vi "CRYSet Control Caption and Text.vi"(8 "Tooltip":string, 9 "Control Type":string, 10 "Caption":string, 11 "Control reference In":refnum<vi>) -> (3 "Control reference out":refnum<vi>)   [LabVIEW 2013]
uses:
  CRYMainGlobal.vi
panel:
  out "error out":errorcluster
  in  "Interpret as Unicode (T)":bool
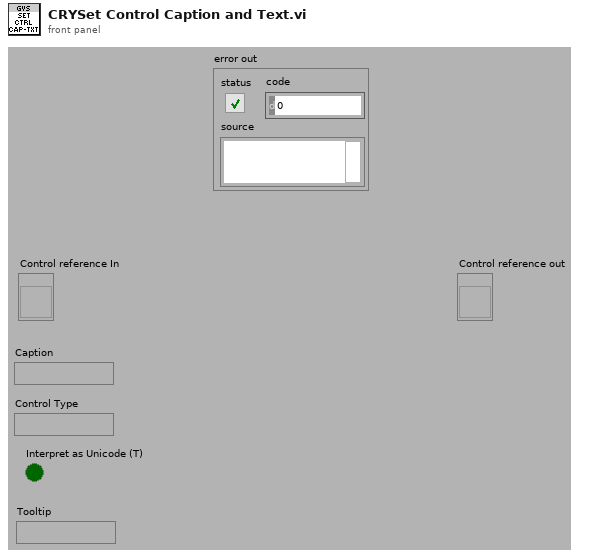
[diagram p1: front panel]
types:
  T1 = enum32{"English", "Chinese", "Korean", "Japanese", "Russian", "Chinese traditional"}
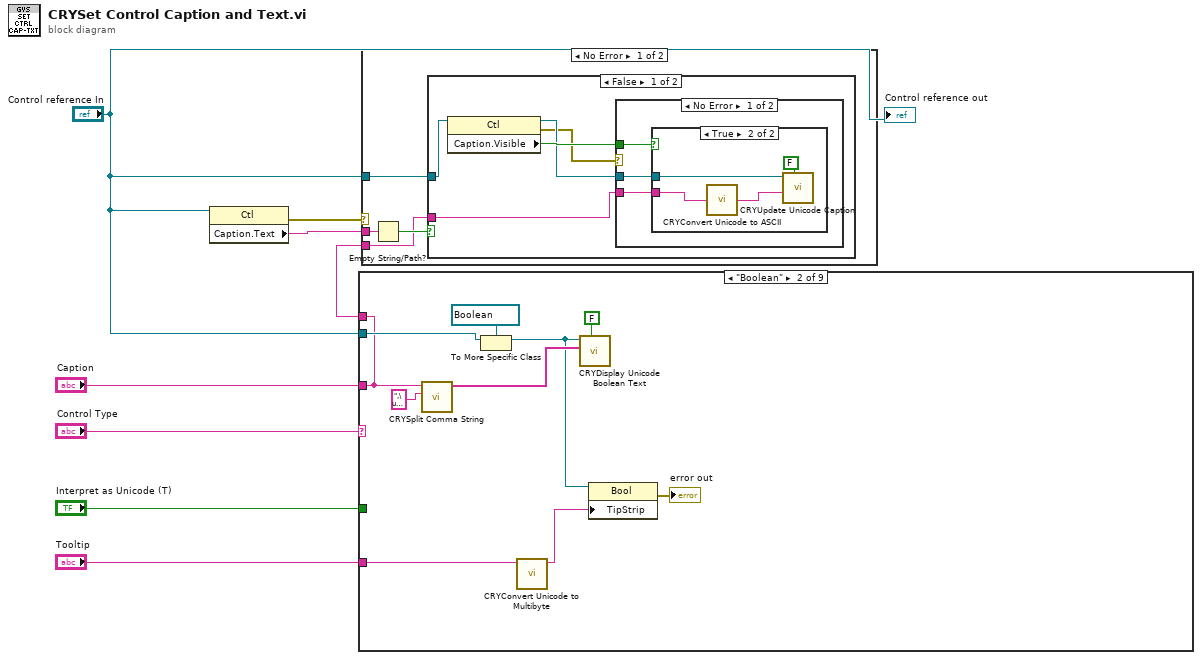
[diagram p0: block diagram]
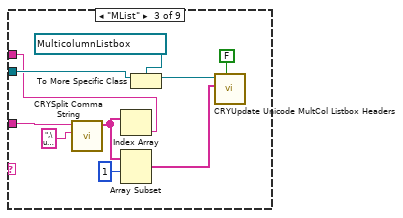
[diagram p7: hidden frame]
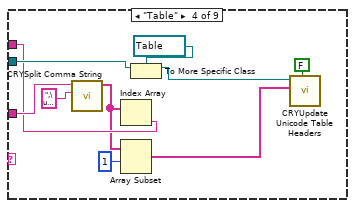
[diagram p8: hidden frame]
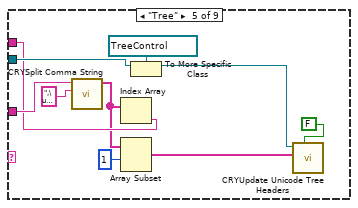
[diagram p9: hidden frame]
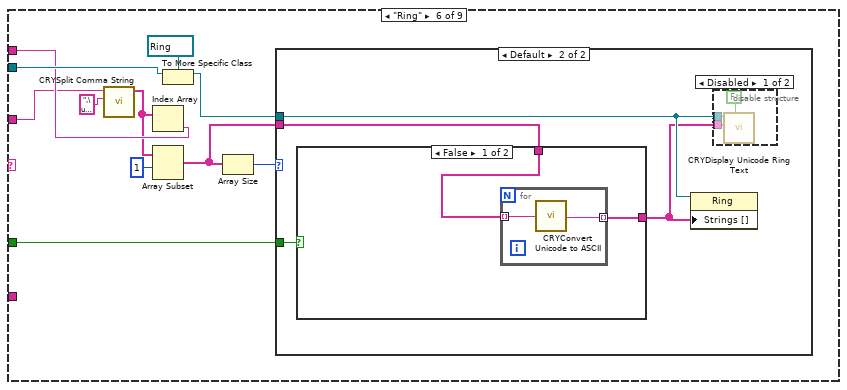
[diagram p10: hidden frame]
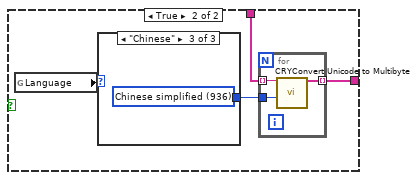
[diagram p12: hidden frame]
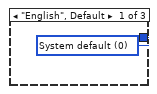
[diagram p13: hidden frame]
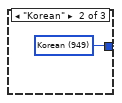
[diagram p14: hidden frame]
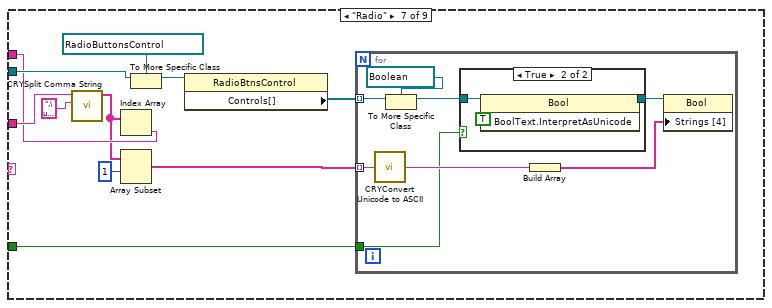
[diagram p16: hidden frame]
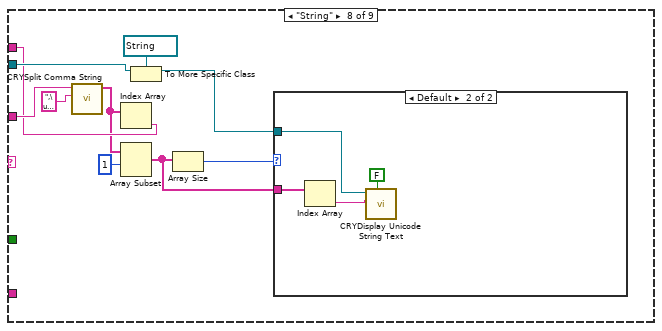
[diagram p18: hidden frame]
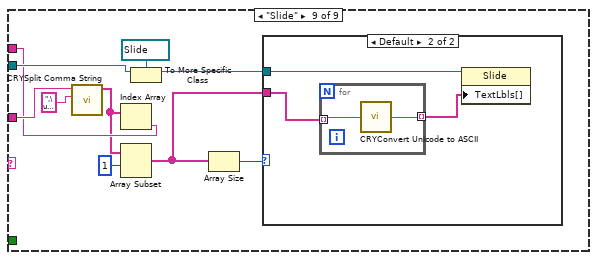
[diagram p20: hidden frame]
diagram:
  n1 = property class="Ctl"(reference="Control reference In") -> (error out=w3:errorcluster, "Caption.Text"=w8:string)  [unwired: 1 in, 1 out]
  n2 = case shown="\"Boolean\"" "Control Type" {
    tunnel: "Control reference In" -> [_ w18 w29 w39 w49 w60 w92 w114 w128]
    tunnel: "Caption" -> [w9 w14 w27 w38 w48 w51 w91 w113 w127]
    tunnel: [w9 w14 w23 w36 w46 w59 w90 w112 w125] -> w4
    tunnel: "Interpret as Unicode (T)" -> [_ _ _ _ _ w50 w82 _ _]
    tunnel: "Tooltip" -> [_ w11 _ _ _ _ _ _ _]
    frame Default {
    }
    frame "Boolean" {
      n3 = call "CRYSplit Comma String.vi"("sSplit Letter"=",\u0000" ("Label.Text"), "sData Out"=w14) -> ("Array"=w16:string[])  [unwired: 9 in]
      n4 = To More Specific Class(target class=refnum<vi> refnum ("Tab Control"), reference=w18) -> (specific class reference=w13:refnum<vi>)  [unwired: 1 in, 1 out]
      n5 = call "CRYConvert Unicode to Multibyte.vi"("Unicode String"=w11) -> ("Multibyte string"=w10:string)  [unwired: 9 in, 1 out]
      n6 = call "CRYDisplay Unicode Boolean Text.vi"("Interpret as Unicode (T)"=FALSE, "Boolean Texts [4]"=w16, "Boolean Reference"=w13) -> ()  [unwired: 5 in, 2 out]
      n7 = property class="Bool"(reference=w13, "TipStrip"=w10) -> (error out=→"error out":errorcluster)  [unwired: 1 in, 1 out]
    }
    frame "MList" {
      n8 = call "CRYSplit Comma String.vi"("sSplit Letter"=",\u0000" ("Label.Text"), "sData Out"=w27) -> ("Array"=w22:string[])  [unwired: 9 in]
      n9 = Index Array(array=w22) -> (element=w23:string)  [unwired: 1 in]
      n10 = Array Subset(array=w22, index=1) -> (w20:string[])  [unwired: 1 in]
      n11 = To More Specific Class(target class=refnum<vi> refnum ("Multicolumn Listbox Ref"), reference=w29) -> (specific class reference=w24:refnum<vi>)  [unwired: 1 in, 1 out]
      n12 = call "CRYUpdate Unicode MultCol Listbox Headers.vi"("Interpret as Unicode (T)"=FALSE, "Column Headers[]"=w20, "Multicolumn Listbox Ref"=w24) -> ()  [unwired: 7 in, 2 out]
    }
    frame "Table" {
      n13 = call "CRYSplit Comma String.vi"("sSplit Letter"=",\u0000" ("Label.Text"), "sData Out"=w38) -> ("Array"=w35:string[])  [unwired: 9 in]
      n14 = Index Array(array=w35) -> (element=w36:string)  [unwired: 1 in]
      n15 = Array Subset(array=w35, index=1) -> (w32:string[])  [unwired: 1 in]
      n16 = To More Specific Class(target class=refnum<vi> refnum ("Table Ref"), reference=w39) -> (specific class reference=w31:refnum<vi>)  [unwired: 1 in, 1 out]
      n17 = call "CRYUpdate Unicode Table Headers.vi"("Interpret as Unicode (T)"=FALSE, "Column Headers[]"=w32, "Table Ref"=w31) -> ()  [unwired: 7 in, 2 out]
    }
    frame "Tree" {
      n18 = call "CRYSplit Comma String.vi"("sSplit Letter"=",\u0000" ("Label.Text"), "sData Out"=w48) -> ("Array"=w45:string[])  [unwired: 9 in]
      n19 = Index Array(array=w45) -> (element=w46:string)  [unwired: 1 in]
      n20 = Array Subset(array=w45, index=1) -> (w43:string[])  [unwired: 1 in]
      n21 = To More Specific Class(target class=refnum<vi> refnum ("Table Ref"), reference=w49) -> (specific class reference=w40:refnum<vi>)  [unwired: 1 in, 1 out]
      n22 = call "CRYUpdate Unicode Tree Headers.vi"("Interpret as Unicode (T)"=FALSE, "Column Headers[]"=w43, "Tree Ref"=w40) -> ()  [unwired: 7 in, 2 out]
    }
    frame "Ring" {
      n23 = call "CRYSplit Comma String.vi"("sSplit Letter"=",\u0000" ("Label.Text"), "sData Out"=w51) -> ("Array"=w57:string[])  [unwired: 9 in]
      n24 = Index Array(array=w57) -> (element=w59:string)  [unwired: 1 in]
      n25 = Array Subset(array=w57, index=1) -> (w53:string[])  [unwired: 1 in]
      n26 = To More Specific Class(target class=refnum<vi> refnum ("Ring Control Ref"), reference=w60) -> (specific class reference=w54:refnum<vi>)  [unwired: 1 in, 1 out]
      n27 = Array Size(array=w53) -> (size(s)=w52:i32)
      n28 = case shown="Default" w52 {
        tunnel: w54 -> [_ w63]
        tunnel: w53 -> [_ w64]
        tunnel: w50 -> [_ w61]
        frame 0 {
        }
        frame Default {
          n29 = case shown="False" w61 {
            tunnel: w64 -> [w66 w70]
            tunnel: [w65 w69] -> w62
            frame False {
              n30 = for {
                tunnel: w66 -> [w68] mode=indexing
                tunnel: [w67] -> w65 mode=indexing
                n31 = call "CRYConvert Unicode to ASCII.vi"("Unicode"=w68) -> ("ASCII"=w67:string)  [unwired: 4 in]
              }
            }
            frame True {
              n32 = global read "CRYMainGlobal.vi" "Language"() -> (w72:T1)
              n33 = case shown="\"Chinese\"" w72 {
                tunnel: [w76 w77 w78] -> w71
                frame "English", Default {
                  w76 = u32 0 items=["System default"=0, "Latin-1"=1252, "Japanese"=932, "Korean"=949, "Chinese simplified"=936, "Chinese traditional"=950, "Central Europe"=1250, "Cyrillic"=1251, "Greek"=1253, "Turkish"=1254, "Hebrew"=1255, "Arabic"=1256, "Baltic"=1257, "Thai"=874, "Vietnamese"=783, "UTF8"=65001, "UTF-7"=65000] ("Code Page")
                }
                frame "Korean" {
                  w77 = u32 949 items=["System default"=0, "Latin-1"=1252, "Japanese"=932, "Korean"=949, "Chinese simplified"=936, "Chinese traditional"=950, "Central Europe"=1250, "Cyrillic"=1251, "Greek"=1253, "Turkish"=1254, "Hebrew"=1255, "Arabic"=1256, "Baltic"=1257, "Thai"=874, "Vietnamese"=783, "UTF8"=65001, "UTF-7"=65000] ("Code Page")
                }
                frame "Chinese" {
                  w78 = u32 936 items=["System default"=0, "Latin-1"=1252, "Japanese"=932, "Korean"=949, "Chinese simplified"=936, "Chinese traditional"=950, "Central Europe"=1250, "Cyrillic"=1251, "Greek"=1253, "Turkish"=1254, "Hebrew"=1255, "Arabic"=1256, "Baltic"=1257, "Thai"=874, "Vietnamese"=783, "UTF8"=65001, "UTF-7"=65000] ("Code Page")
                }
              }
              n34 = for {
                tunnel: w70 -> [w75] mode=indexing
                tunnel: [w74] -> w69 mode=indexing
                tunnel: w71 -> [w73]
                n35 = call "CRYConvert Unicode to Multibyte.vi"("Code Page"=w73, "Unicode String"=w75) -> ("Multibyte string"=w74:string)  [unwired: 8 in, 1 out]
              }
            }
          }
          n36 = property class="Ring"(reference=w63, "Strings []"=w62) -> ()  [unwired: 1 in, 2 out]
          n37 = disable-structure shown="Disabled" {
            disable-tunnel: w63 -> [w80 _]
            disable-tunnel: w62 -> [w79 _]
            frame Disabled {
              n38 = call "CRYDisplay Unicode Ring Text.vi"("Interpret as Unicode (T)"=FALSE, "Ring Texts"=w79, "Ring Control Ref"=w80) -> ()  [unwired: 5 in, 2 out]
            }
            frame Enabled {
            }
          }
        }
      }
    }
    frame "Radio" {
      n39 = call "CRYSplit Comma String.vi"("sSplit Letter"=",\u0000" ("Label.Text"), "sData Out"=w91) -> ("Array"=w88:string[])  [unwired: 9 in]
      n40 = Index Array(array=w88) -> (element=w90:string)  [unwired: 1 in]
      n41 = Array Subset(array=w88, index=1) -> (w83:string[])  [unwired: 1 in]
      n42 = To More Specific Class(target class=refnum<vi> refnum ("Radio Buttons"), reference=w92) -> (specific class reference=w85:refnum<vi>)  [unwired: 1 in, 1 out]
      n43 = property class="RadioBtnsControl"(reference=w85) -> ("Controls[]"=w84:refnum<vi>[])  [unwired: 1 in, 2 out]
      n44 = for {
        tunnel: w84 -> [w99] mode=indexing
        tunnel: w83 -> [w95] mode=indexing
        tunnel: w82 -> [w93]
        n45 = call "CRYConvert Unicode to ASCII.vi"("Unicode"=w95) -> ("ASCII"=w94:string)  [unwired: 4 in]
        n46 = To More Specific Class(target class=refnum<vi> refnum ("Radio Selection 2"), reference=w99) -> (specific class reference=w97:refnum<vi>)  [unwired: 1 in, 1 out]
        n47 = case shown="True" w93 {
          tunnel: w97 -> [w101 w104]
          tunnel: [w101 w102] -> w96
          frame False {
          }
          frame True {
            n48 = property class="Bool"(reference=w104, "BoolText.InterpretAsUnicode"=TRUE ("Boolean Text.Interpret As Unicode")) -> (reference out=w102:refnum<vi>)  [unwired: 1 in, 1 out]
          }
        }
        n49 = Build Array(w94) -> (w98:string[])
        n50 = property class="Bool"(reference=w96, "Strings [4]"=w98) -> ()  [unwired: 1 in, 2 out]
      }
    }
    frame "String" {
      n51 = call "CRYSplit Comma String.vi"("sSplit Letter"=",\u0000" ("Label.Text"), "sData Out"=w113) -> ("Array"=w110:string[])  [unwired: 9 in]
      n52 = Index Array(array=w110) -> (element=w112:string)  [unwired: 1 in]
      n53 = Array Subset(array=w110, index=1) -> (w105:string[])  [unwired: 1 in]
      n54 = To More Specific Class(target class=refnum<vi> refnum ("Radio Buttons"), reference=w114) -> (specific class reference=w106:refnum<vi>)  [unwired: 1 in, 1 out]
      n55 = Array Size(array=w105) -> (size(s)=w107:i32)
      n56 = case shown="Default" w107 {
        tunnel: w106 -> [_ w117]
        tunnel: w105 -> [_ w118]
        frame 0 {
        }
        frame Default {
          n57 = Index Array(array=w118) -> (element=w116:string)  [unwired: 1 in]
          n58 = call "CRYDisplay Unicode String Text.vi"("Interpret as Unicode (T)"=FALSE, "String Value"=w116, "String Control Reference"=w117) -> ()  [unwired: 5 in, 2 out]
        }
      }
    }
    frame "Slide" {
      n59 = call "CRYSplit Comma String.vi"("sSplit Letter"=",\u0000" ("Label.Text"), "sData Out"=w127) -> ("Array"=w124:string[])  [unwired: 9 in]
      n60 = Index Array(array=w124) -> (element=w125:string)  [unwired: 1 in]
      n61 = Array Subset(array=w124, index=1) -> (w120:string[])  [unwired: 1 in]
      n62 = To More Specific Class(target class=refnum<vi> refnum ("Scale 2"), reference=w128) -> (specific class reference=w121:refnum<vi>)  [unwired: 1 in, 1 out]
      n63 = Array Size(array=w120) -> (size(s)=w119:i32)
      n64 = case shown="Default" w119 {
        tunnel: w121 -> [_ w131]
        tunnel: w120 -> [_ w130]
        frame 0 {
        }
        frame Default {
          n65 = for {
            tunnel: w130 -> [w133] mode=indexing
            tunnel: [w132] -> w129 mode=indexing
            n66 = call "CRYConvert Unicode to ASCII.vi"("Unicode"=w133) -> ("ASCII"=w132:string)  [unwired: 4 in]
          }
          n67 = property class="Slide"(reference=w131, "TextLbls[]"=w129) -> ()  [unwired: 1 in, 2 out]
        }
      }
    }
  }
  n68 = case shown="No Error" w3 {
    tunnel: w8 -> [w136 _]
    tunnel: "Control reference In" -> [w135 _]
    tunnel: w4 -> [w134 _]
    frame No Error {
      n69 = Empty String/Path?(string/path=w136) -> (empty?=w137:bool)
      n70 = case shown="False" w137 {
        tunnel: w135 -> [w140 _]
        tunnel: w134 -> [w139 _]
        frame False {
          n71 = property class="Ctl"(reference=w140) -> (error out=w138:errorcluster, "Caption.Visible"=w141:bool)  [unwired: 1 in, 1 out]
          n72 = case shown="No Error" w138 {
            tunnel: w141 -> [w144 _]
            tunnel: w140 -> [w143 _]
            tunnel: w139 -> [w142 _]
            frame No Error {
              n73 = case shown="True" w144 {
                tunnel: w143 -> [_ w148]
                tunnel: w142 -> [_ w146]
                frame False {
                }
                frame True {
                  n74 = call "CRYConvert Unicode to ASCII.vi"("Unicode"=w146) -> ("ASCII"=w145:string)  [unwired: 4 in]
                  n75 = call "CRYUpdate Unicode Caption.vi"("Interpret as Unicode (T)"=FALSE, "Caption"=w145, "Control Reference"=w148) -> ()  [unwired: 5 in, 2 out]
                }
              }
            }
            frame Error {
            }
          }
        }
        frame True {
        }
      }
    }
    frame Error {
    }
  }
  "Control reference out" <- "Control reference In"
